vi "DisplayPanel.vi"() -> ()   [LabVIEW 2015]
uses:
  <vilib>/picture/picture.llb/imagedata.ctl
  MvLVLib/MvCameraControl.lvlib
panel:
  out "GenTLDevInfoArray":T1(array[cluster])
  out "GenTLIfInfoArray":T2(array[cluster])
  in  "Refresh Interaces":bool
  in  "Interface List":u16(ring) items=["[GenTL] GEVGenTL Interface Module"]
  in  "pConvertInfo In":T3
  out "PixelFormat":u32
  out "handle out":u64
  in  "handle":u64
  in  "Rectangle":T4
  in  "image data":T5 caption="图像数据"
  out "Picture":picture
  out "PayloadSize":u32
  out "pFrameInfoEx out":T6
  out "nHeight":u32
  out "nWidth":u32
  out "Acquisision Flag":bool
  in  "Trigger Mode":bool
  in  "Continuous":bool
  out "打开标志":bool
  in  "stop":bool
  in  "Trigger Once":bool
  in  "Stop":bool
  in  "Start":bool
  in  "Open Device":bool
  in  "Close Device":bool
  in  "error in (no error) 2":errorcluster caption="错误输入（无错误）"
  in  "Refresh Devices":bool
  in  "Device List":u16(ring) items=["[GenTL] DJFL MV-DB1608-05C-H-S(00202009042)", "[GenTL] SmartCamera_wmr MV-ID6089M-00C-NNG(00236610549)", "[GenTL] Don't Connect MV-CA013-20GM(00643989004)", "[GenTL] zyb MV-CA020-20GM(00683551272)", "[GenTL] 二维 MV-CA060-11GM(00815677386)", "[GenTL] ZLR MV-CE120-10GC(00C87836158)", "[GenTL] 132中文 MV-CA013-20GC(00C91585464)", "[GenTL] BionCamera1 MV-DB1308-05H(00D27684654)", "[GenTL] SZP 349Camera MV-ID6200M-00C-NNG(00D57564216)", "[GenTL] 8 MV-ID6200M-00C-NNG(00D75479067)", "[GenTL]  MV-DL2025-04H-H(00E35281809)", "[GenTL]  MV-DL2025-04H-H(00E47782357)", "[GenTL] smartcamera_ff MV-ID6200M-00C-NNG(00F36543614)", "[GenTL] left MV-ID6200M-00C-NNG(00F62465456)", "[GenTL]  EX-YTO-GM(00G02928059)", "[GenTL] BaseX86_1 MV-SI612-06GM(C12222347)", "[GenTL] CS060_csj MV-CS060-10GC-PRO(E55846631)", "[GenTL] zxc_SC_3016C MV-SC3016C-12M-WBN(G07812386)", "[GenTL] zxc_SC_2004EM MV-SC2004EM-06S-WBN(G32318424)"]
  # "Initialize"
  # "Acquisition"
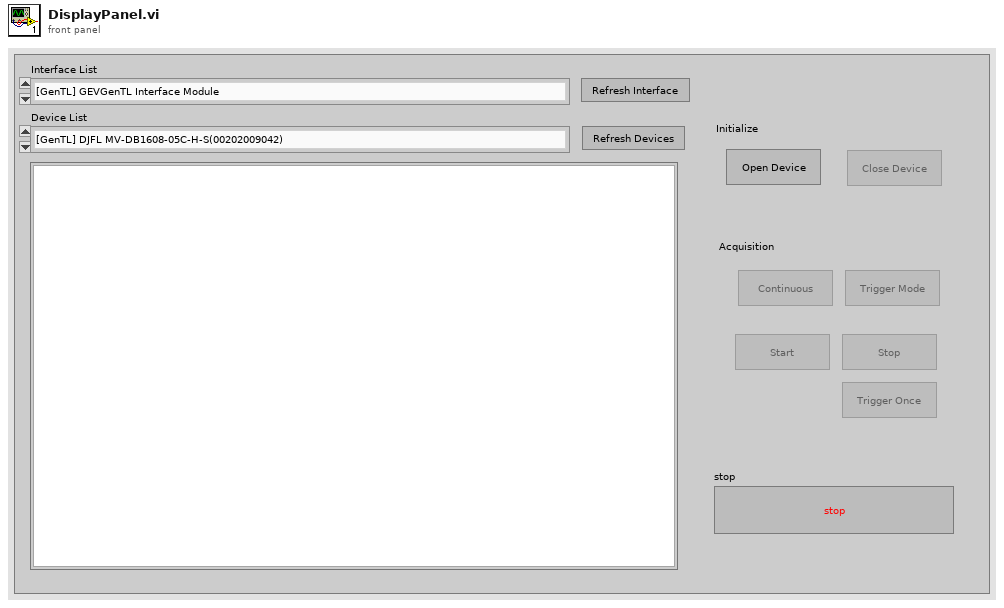
[diagram p1: front panel]
types:
  T1 = cluster{"chInterfaceID":string, "chDeviceID":string, "chVendorName":string, "chModelName":string, "chTLType":string, "chDisplayName":string, "chUserDefinedName":string, "chSerialNumber":string, "chDeviceVersion":string, "nCtiIndex":u32, "nReserved[0]":u32, "nReserved[1]":u32, "nReserved[2]":u32, "nReserved[3]":u32, "nReserved[4]":u32, "nReserved[5]":u32, "nReserved[6]":u32, "nReserved[7]":u32}[]
  T2 = cluster{"chInterfaceID":string, "chTLType":string, "chDisplayName":string, "nCtiIndex":u32, "nReserved[0]":u32, "nReserved[1]":u32, "nReserved[2]":u32, "nReserved[3]":u32, "nReserved[4]":u32, "nReserved[5]":u32, "nReserved[6]":u32, "nReserved[7]":u32}[]
  T3 = cluster{"nWidth":u16, "nHeight":u16, "enSrcPixelType":u32, "nSrcDataLen":u32, "enDstPixelType":u32, "nDstLen":u32, "nDstBufferSize":u32, "nRes0":u32, "nRes1":u32, "nRes2":u32, "nRes3":u32}
  T4 = cluster{"left":i16, "top":i16, "right":i16, "bottom":i16}
  T5 = typedef "imagedata.ctl" = cluster{"image type":i32, "image depth":i32, "image":u8[], "mask":u8[], "colors":u32[], "Rectangle":cluster{"left":i16, "top":i16, "right":i16, "bottom":i16}}
  T6 = cluster{"nWidth":u16, "nHeight":u16, "enPixelType":i32, "nFrameNum":u32, "nDevTimeStampHigh":u32, "nDevTimeStampLow":u32, "nReserved0":u32, "nHostTimeStamp":i64, "nFrameLen":u32, "nSecondCount]":u32, "nCycleCount":u32, "nCycleOffset":u32, "fGain":u32, "fExposureTime":u32, "nAverageBrightness":u32, "nRed":u32, "nGreen":u32, "nBlue":u32, "nFrameCounter":u32, "nTriggerIndex":u32, "nInput":u32, "nOutput":u32, "nOffsetX":u32, "nOffsetY":u32, "nReserved[0]":u32, "nReserved[1]":u32, "nReserved[2]":u32, "nReserved[3]":u32, "nReserved[4]":u32, "nReserved[5]":u32, "nReserved[6]":u32, "nReserved[7]":u32, "nReserved[8]":u32, "nReserved[9]":u32, "nReserved[10]":u32, "nReserved[11]":u32, "nReserved[12]":u32, "nReserved[13]":u32, "nReserved[14] 10":u32, "nReserved[15] 11":u32, "nReserved[16] 12":u32, "nReserved[17] 13":u32, "nReserved[18] 14":u32, "nReserved[19] 15":u32, "nReserved[20] 16":u32, "nReserved[21] 17":u32, "nReserved[22] 18":u32, "nReserved[23] 19":u32, "nReserved[24] 20":u32, "nReserved[25] 21":u32, "nReserved[26] 22":u32, "nReserved[27] 23":u32, "nReserved[28] 24":u32, "nReserved[29] 25":u32, "nReserved[30] 26":u32, "nReserved[31] 27":u32, "nReserved[32] 28":u32, "nReserved[33] 29":u32, "nReserved[34] 30":u32, "nReserved[35] 31":u32, "nReserved[36] 32":u32, "nReserved[37] 33":u32, "nReserved[38] 34":u32, "nReserved[39] 35":u32, "nReserved[40] 36":u32}
  T7 = enum8{"Enabled", "Disabled", "Disabled and Grayed Out"}
  T8 = cluster{"nCurValue":u32, "nMax":u32, "nMin":u32, "nInc":u32, "nReserved[0]":u32, "nReserved[1]":u32, "nReserved[2]":u32, "nReserved[3]":u32}
  T9 = cluster{"nCurValue":u32, "nSupportedNum":u32, "nSupportValue[0]":u32, "nSupportValue[1]":u32, "nSupportValue[2]":u32, "nSupportValue[3]":u32, "nSupportValue[4]":u32, "nSupportValue[5]":u32, "nSupportValue[6]":u32, "nSupportValue[7]":u32, "nSupportValue[8]":u32, "nSupportValue[9]":u32, "nSupportValue[10]":u32, "nSupportValue[11]":u32, "nSupportValue[12]":u32, "nSupportValue[13]":u32, "nSupportValue[14]":u32, "nSupportValue[15]":u32, "nSupportValue[16]":u32, "nSupportValue[17]":u32, "nSupportValue[18]":u32, "nSupportValue[19]":u32, "nSupportValue[20]":u32, "nSupportValue[21]":u32, "nSupportValue[22]":u32, "nSupportValue[23]":u32, "nSupportValue[24]":u32, "nSupportValue[25]":u32, "nSupportValue[26]":u32, "nSupportValue[27]":u32, "nSupportValue[28]":u32, "nSupportValue[29]":u32, "nSupportValue[30]":u32, "nSupportValue[31]":u32, "nSupportValue[32]":u32, "nSupportValue[33]":u32, "nSupportValue[34]":u32, "nSupportValue[35]":u32, "nSupportValue[36]":u32, "nSupportValue[37]":u32, "nSupportValue[38]":u32, "nSupportValue[39]":u32, "nSupportValue[40]":u32, "nSupportValue[41]":u32, "nSupportValue[42]":u32, "nSupportValue[43]":u32, "nSupportValue[44]":u32, "nSupportValue[45]":u32, "nSupportValue[46]":u32, "nSupportValue[47]":u32, "nSupportValue[48]":u32, "nSupportValue[49]":u32, "nSupportValue[50]":u32, "nSupportValue[51]":u32, "nSupportValue[52]":u32, "nSupportValue[53]":u32, "nSupportValue[54]":u32, "nSupportValue[55]":u32, "nSupportValue[56]":u32, "nSupportValue[57]":u32, "nSupportValue[58]":u32, "nSupportValue[59]":u32, "nSupportValue[60]":u32, "nSupportValue[61]":u32, "nSupportValue[62]":u32, "nSupportValue[63]":u32, "nReserved[0]":u32, "nReserved[1]":u32, "nReserved[2]":u32, "nReserved[3]":u32}
  T10 = cluster{"chInterfaceID":string, "chTLType":string, "chDisplayName":string, "nCtiIndex":u32, "nReserved[0]":u32, "nReserved[1]":u32, "nReserved[2]":u32, "nReserved[3]":u32, "nReserved[4]":u32, "nReserved[5]":u32, "nReserved[6]":u32, "nReserved[7]":u32}
  T11 = cluster{"chInterfaceID":string, "chDeviceID":string, "chVendorName":string, "chModelName":string, "chTLType":string, "chDisplayName":string, "chUserDefinedName":string, "chSerialNumber":string, "chDeviceVersion":string, "nCtiIndex":u32, "nReserved[0]":u32, "nReserved[1]":u32, "nReserved[2]":u32, "nReserved[3]":u32, "nReserved[4]":u32, "nReserved[5]":u32, "nReserved[6]":u32, "nReserved[7]":u32}
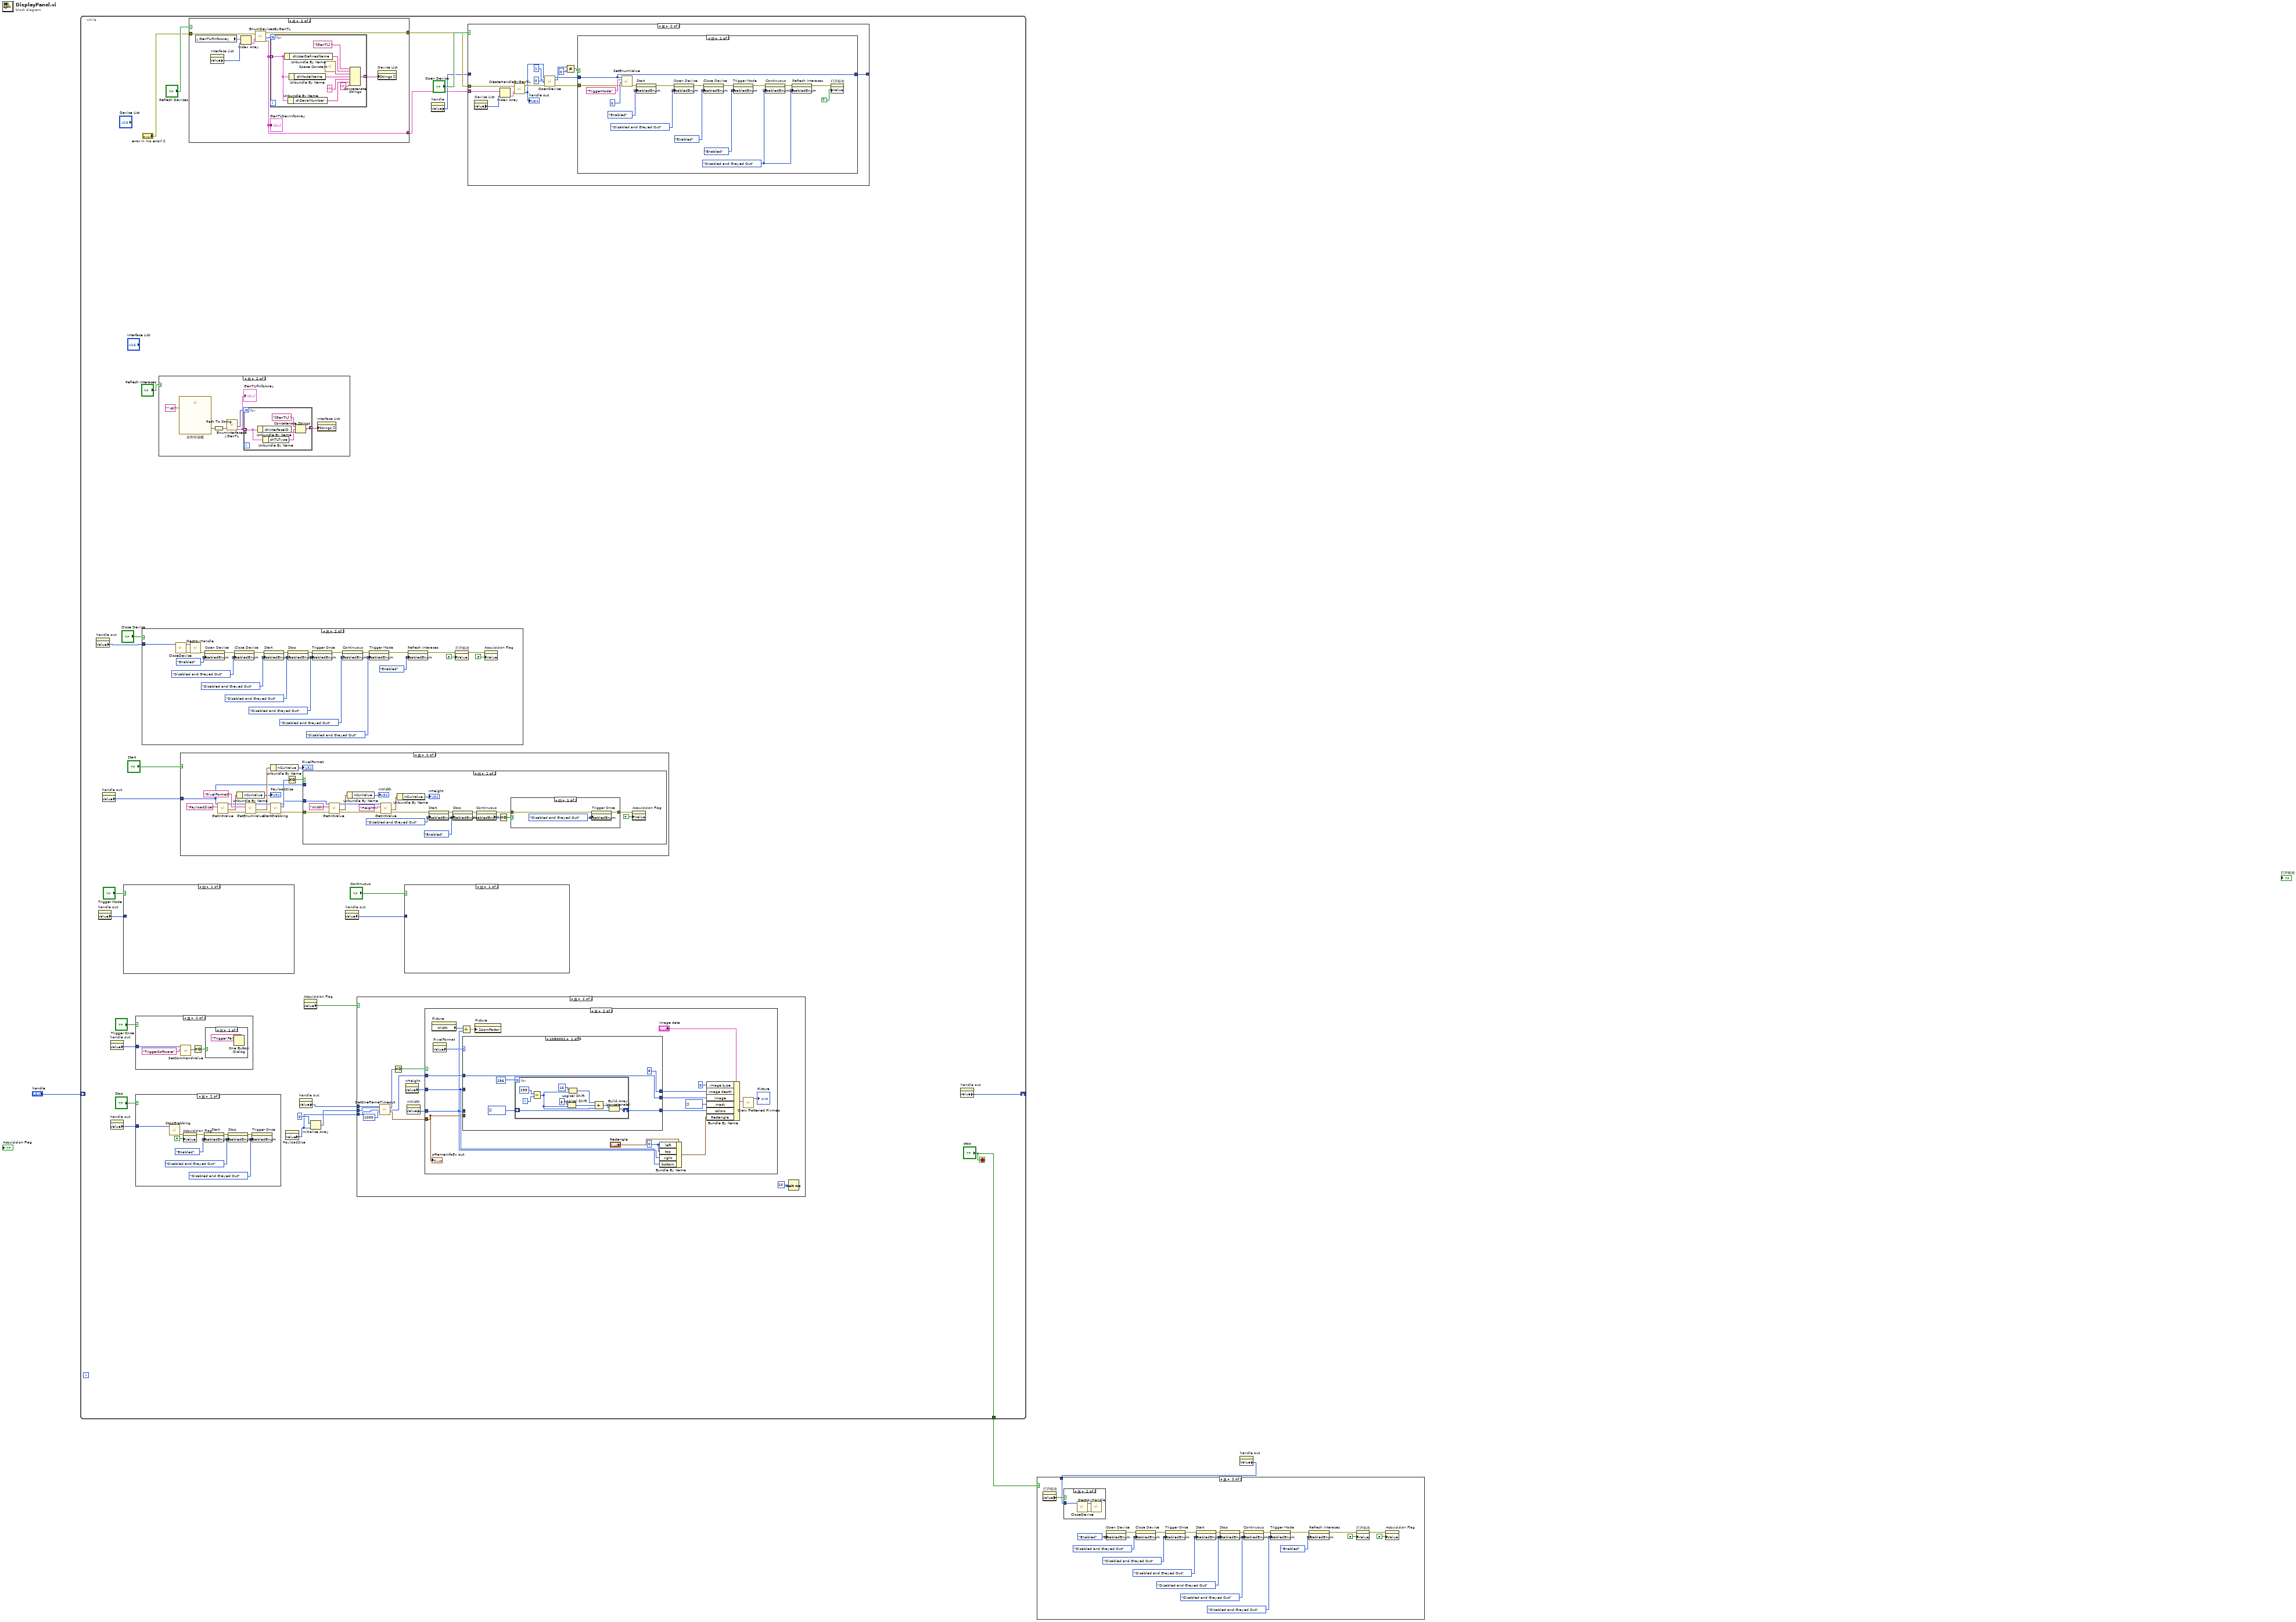
[diagram p0: block diagram]
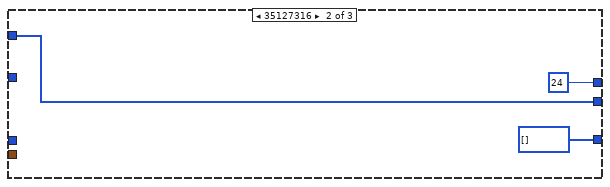
[diagram p7: hidden frame]
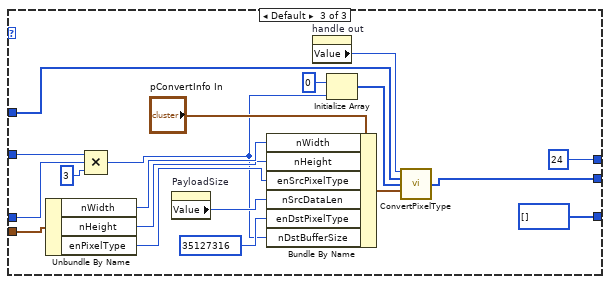
[diagram p8: hidden frame]
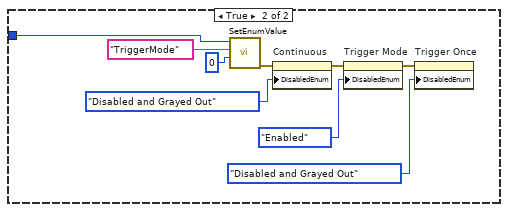
[diagram p10: hidden frame]
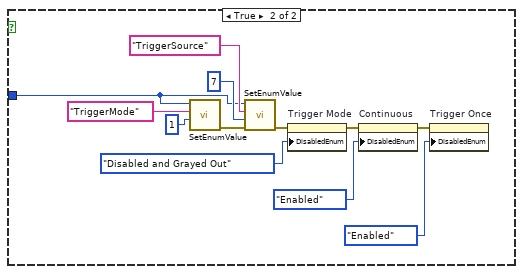
[diagram p11: hidden frame]
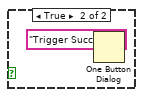
[diagram p13: hidden frame]
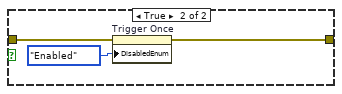
[diagram p15: hidden frame]
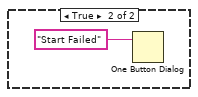
[diagram p16: hidden frame]
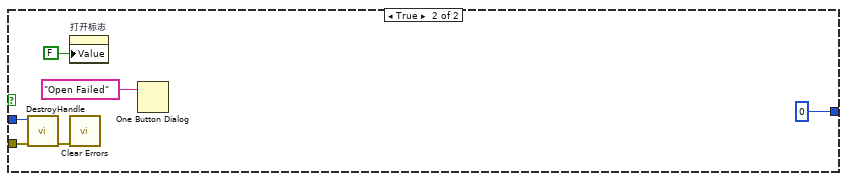
[diagram p19: hidden frame]
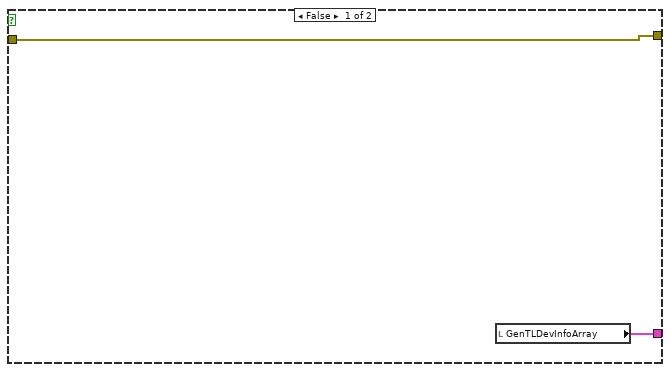
[diagram p20: hidden frame]
diagram:
  n1 = while {
    tunnel: ["stop"] -> w3
    shift-right: [w17] -> _
    shift-left: "handle" -> [_]
    stop <- "stop" stop-if-true
    n2 = property on="handle out" class="DigNum (严格)"() -> ("Value"=w15:u64)  [unwired: 2 in, 2 out]
    n3 = property on="handle out" class="DigNum (严格)"() -> ("Value"=w10:u64)  [unwired: 2 in, 2 out]
    n4 = property on="handle out" class="DigNum (严格)"() -> ("Value"=w11:u64)  [unwired: 2 in, 2 out]
    n5 = property on="handle out" class="DigNum (严格)"() -> ("Value"=w14:u64)  [unwired: 2 in, 2 out]
    n6 = property on="handle out" class="DigNum (严格)"() -> ("Value"=w13:u64)  [unwired: 2 in, 2 out]
    n7 = case shown="假" "Trigger Mode" {
      tunnel: w10 -> [_ w125]
      frame False {
      }
      frame True {
        n8 = call "SetEnumValue.vi"("nValue"=u32 1, "strKey"="TriggerMode", "handle"=w125) -> ("error out"=w131:errorcluster)  [unwired: 6 in, 2 out]
        n9 = call "SetEnumValue.vi"("error in (no error)"=w131, "nValue"=u32 7, "strKey"="TriggerSource", "handle"=w125) -> ("error out"=w130:errorcluster)  [unwired: 5 in, 2 out]
        n10 = property on="Trigger Mode" class="Bool"(error in=w130, "DisabledEnum"=T7."Disabled and Grayed Out" ("禁用")) -> (error out=w129:errorcluster)  [unwired: 1 in, 1 out]
        n11 = property on="Continuous" class="Bool"(error in=w129, "DisabledEnum"=T7."Enabled" ("禁用")) -> (error out=w127:errorcluster)  [unwired: 1 in, 1 out]
        n12 = property on="Trigger Once" class="Bool"(error in=w127, "DisabledEnum"=T7."Enabled" ("禁用")) -> ()  [unwired: 1 in, 2 out]
      }
    }
    n13 = case shown="真" "Trigger Once" {
      tunnel: w14 -> [_ w140]
      frame False {
      }
      frame True {
        n14 = call "SetCommandValue.vi"("strValue"="TriggerSoftware", "handle"=w140) -> ("function return"=w138:i32)  [unwired: 7 in, 2 out]
        n15 = Equal To 0?(x=w138) -> (x = 0?=w137:bool)
        n16 = case shown="假" w137 {
          frame False {
            n17 = One Button Dialog(message="Trigger Failed") -> ()  [unwired: 1 in, 1 out]
          }
          frame True {
            n18 = One Button Dialog(message="Trigger Success") -> ()  [unwired: 1 in, 1 out]
          }
        }
      }
    }
    n19 = case shown="真" "Stop" {
      tunnel: w13 -> [_ w115]
      frame False {
      }
      frame True {
        n20 = call "StopGrabbing.vi"("handle"=w115) -> ("error out"=w114:errorcluster)  [unwired: 8 in, 2 out]
        n21 = property on="Acquisision Flag" class="Bool (严格)"(error in=w114, "Value"=FALSE ("采集标志")) -> (error out=w109:errorcluster)  [unwired: 1 in, 1 out]
        n22 = property on="Start" class="Bool"(error in=w109, "DisabledEnum"=T7."Enabled" ("禁用")) -> (error out=w108:errorcluster)  [unwired: 1 in, 1 out]
        n23 = property on="Stop" class="Bool"(error in=w108, "DisabledEnum"=T7."Disabled and Grayed Out" ("禁用")) -> (error out=w107:errorcluster)  [unwired: 1 in, 1 out]
        n24 = property on="Trigger Once" class="Bool"(error in=w107, "DisabledEnum"=T7."Disabled and Grayed Out" ("禁用")) -> ()  [unwired: 1 in, 2 out]
      }
    }
    n25 = case shown="真" "Close Device" {
      tunnel: w15 -> [_ w190]
      frame False {
      }
      frame True {
        n26 = call "CloseDevice.vi"("handle"=w190) -> ("error out"=w192:errorcluster, "handle out"=w189:u64)  [unwired: 8 in, 1 out]
        n27 = call "DestroyHandle.vi"("error in (no error)"=w192, "handle"=w189) -> ("error out"=w191:errorcluster)  [unwired: 8 in, 1 out]
        n28 = property on="Open Device" class="Bool"(error in=w191, "DisabledEnum"=T7."Enabled" ("禁用")) -> (error out=w203:errorcluster)  [unwired: 1 in, 1 out]
        n29 = property on="Close Device" class="Bool"(error in=w203, "DisabledEnum"=T7."Disabled and Grayed Out" ("禁用")) -> (error out=w202:errorcluster)  [unwired: 1 in, 1 out]
        n30 = property on="Start" class="Bool"(error in=w202, "DisabledEnum"=T7."Disabled and Grayed Out" ("禁用")) -> (error out=w201:errorcluster)  [unwired: 1 in, 1 out]
        n31 = property on="Stop" class="Bool"(error in=w201, "DisabledEnum"=T7."Disabled and Grayed Out" ("禁用")) -> (error out=w200:errorcluster)  [unwired: 1 in, 1 out]
        n32 = property on="Trigger Once" class="Bool"(error in=w200, "DisabledEnum"=T7."Disabled and Grayed Out" ("禁用")) -> (error out=w197:errorcluster)  [unwired: 1 in, 1 out]
        n33 = property on="Continuous" class="Bool"(error in=w197, "DisabledEnum"=T7."Disabled and Grayed Out" ("禁用")) -> (error out=w196:errorcluster)  [unwired: 1 in, 1 out]
        n34 = property on="Trigger Mode" class="Bool"(error in=w196, "DisabledEnum"=T7."Disabled and Grayed Out" ("禁用")) -> (error out=w187:errorcluster)  [unwired: 1 in, 1 out]
        n35 = property on="Refresh Interaces" class="Bool"(error in=w187, "DisabledEnum"=T7."Enabled" ("禁用")) -> (error out=w186:errorcluster)  [unwired: 1 in, 1 out]
        n36 = property on="打开标志" class="Bool (严格)"(error in=w186, "Value"=FALSE ("打开标志")) -> (error out=w194:errorcluster)  [unwired: 1 in, 1 out]
        n37 = property on="Acquisision Flag" class="Bool (严格)"(error in=w194, "Value"=FALSE ("采集标志")) -> ()  [unwired: 1 in, 2 out]
      }
    }
    n38 = case shown="真" "Refresh Interaces" {
      frame False {
      }
      frame True {
        n39 = call "文件对话框"("pattern (all files)"="*.cti") -> ("selected path"=w34:path)  [unwired: 11 in, 3 out]
        n40 = Path To String(path=w34) -> (string=w33:string)
        n41 = call "EnumInterfacesByGenTL.vi"("strGenTLPath"=w33) -> ("nInterfaceNum"=w31:u32, "pGenTLIfInfoArray"=w32:T2)  [unwired: 1 in, 2 out]
        "GenTLIfInfoArray" <- w32
        n42 = for {
          N: w31 -> [_]
          tunnel: [w40] -> w30 mode=indexing
          tunnel: w32 -> [w37] mode=indexing
          n43 = Unbundle By Name(w37) -> ("chInterfaceID"=w38:string)
          n44 = Unbundle By Name(w37) -> ("chTLType"=w36:string)
          n45 = Concatenate Strings("[GenTL] " ("字符串"), w36, w38) -> (w40:string)
        }
        n46 = property on="Interface List" class="Ring (严格)"("Strings []"=w30) -> ()  [unwired: 2 in, 2 out]
      }
    }
    n47 = case shown="真" "Start" {
      tunnel: w11 -> [_ w147]
      frame False {
      }
      frame True {
        n48 = call "GetIntValue.vi"("strKey"="PayloadSize", "handle"=w147) -> ("error out"=w153:errorcluster, "pIntValue out"=w149:T8, "handle out"=w145:u64)  [unwired: 6 in, 1 out]
        n49 = Unbundle By Name(w149) -> ("nCurValue"=→"PayloadSize":u32)
        n50 = call "GetEnumValue.vi"("error in (no error)"=w153, "strKey"="PixelFormat", "handle"=w145) -> ("error out"=w152:errorcluster, "pEnumValue out"=w154:T9, "handle out"=w144:u64)  [unwired: 5 in, 1 out]
        n51 = Unbundle By Name(w154) -> ("nCurValue"=→"PixelFormat":u32)
        n52 = call "StartGrabbing.vi"("error in (no error)"=w152, "handle"=w144) -> ("error out"=w151:errorcluster, "function return"=w157:i32, "handle out"=w143:u64)  [unwired: 7 in]
        n53 = Not Equal To 0?(x=w157) -> (x != 0?=w156:bool)
        n54 = case shown="假" w156 {
          tunnel: w147 -> [_ _]
          tunnel: w151 -> [w160 _]
          tunnel: w143 -> [w159 _]
          frame False {
            n55 = call "GetIntValue.vi"("error in (no error)"=w160, "strKey"="Width", "handle"=w159) -> ("error out"=w167:errorcluster, "pIntValue out"=w161:T8, "handle out"=w158:u64)  [unwired: 5 in, 1 out]
            n56 = Unbundle By Name(w161) -> ("nCurValue"=→"nWidth":u32)
            n57 = call "GetIntValue.vi"("error in (no error)"=w167, "strKey"="Height", "handle"=w158) -> ("error out"=w166:errorcluster, "pIntValue out"=w164:T8)  [unwired: 5 in, 2 out]
            n58 = Unbundle By Name(w164) -> ("nCurValue"=→"nHeight":u32)
            n59 = property on="Start" class="Bool"(error in=w166, "DisabledEnum"=T7."Disabled and Grayed Out" ("禁用")) -> (error out=w176:errorcluster)  [unwired: 1 in, 1 out]
            n60 = property on="Stop" class="Bool"(error in=w176, "DisabledEnum"=T7."Enabled" ("禁用")) -> (error out=w162:errorcluster)  [unwired: 1 in, 1 out]
            n61 = property on="Continuous" class="Bool"(error in=w162) -> (error out=w172:errorcluster, "DisabledEnum"=w173:T7)  [unwired: 1 in, 1 out]
            n62 = Equal To 0?(x=w173) -> (x = 0?=w174:bool)
            n63 = case shown="假" w174 {
              tunnel: w172 -> [w179 w182]
              tunnel: [w178 w181] -> w171
              frame False {
                n64 = property on="Trigger Once" class="Bool"(error in=w179, "DisabledEnum"=T7."Disabled and Grayed Out" ("禁用")) -> (error out=w178:errorcluster)  [unwired: 1 in, 1 out]
              }
              frame True {
                n65 = property on="Trigger Once" class="Bool"(error in=w182, "DisabledEnum"=T7."Enabled" ("禁用")) -> (error out=w181:errorcluster)  [unwired: 1 in, 1 out]
              }
            }
            n66 = property on="Acquisision Flag" class="Bool (严格)"(error in=w171, "Value"=TRUE ("采集标志")) -> ()  [unwired: 1 in, 2 out]
          }
          frame True {
            n67 = One Button Dialog(message="Start Failed") -> ()  [unwired: 1 in, 1 out]
          }
        }
      }
    }
    n68 = case shown="真" "Refresh Devices" {
      tunnel: [w247 w250] -> w19
      tunnel: "error in (no error) 2" -> [w247 w251]
      tunnel: [w246 w248] -> w4
      frame False {
        n69 = local read "GenTLDevInfoArray"() -> (w246:T1)
      }
      frame True {
        n70 = local read "GenTLIfInfoArray"() -> (w253:T2)
        n71 = property on="Interface List" class="Ring (严格)"() -> ("Value"=w254:u16)  [unwired: 2 in, 2 out]
        n72 = Index Array(array=w253, index=w254) -> (element=w252:T10)
        n73 = call "EnumDevicesByGenTL.vi"("error in (no error)"=w251, "pIFInfo"=w252) -> ("error out"=w250:errorcluster, "nDeviceNum"=w249:u32, "pGenTLDevInfoArray"=w248:T1)  [unwired: 1 out]
        "GenTLDevInfoArray" <- w248
        n74 = for {
          N: w249 -> [_]
          tunnel: [w261] -> w255 mode=indexing
          tunnel: w248 -> [w259] mode=indexing
          n75 = Unbundle By Name(w259) -> ("chUserDefinedName"=w258:string)
          n76 = Unbundle By Name(w259) -> ("chSerialNumber"=w256:string)
          n77 = Unbundle By Name(w259) -> ("chModelName"=w257:string)
          n78 = call <vilib>:"Space Constant.vi"() -> ("String"=w264:string)
          n79 = Concatenate Strings("[GenTL] " ("字符串"), w258, w264, w257, "(" ("字符串"), w256, ")" ("字符串")) -> (w261:string)
        }
        n80 = property on="Device List" class="Ring (严格)"("Strings []"=w255) -> ()  [unwired: 2 in, 2 out]
      }
    }
    n81 = property on="PayloadSize" class="DigNum (严格)"() -> ("Value"=w6:u32)  [unwired: 2 in, 2 out]
    n82 = property on="handle out" class="DigNum (严格)"() -> ("Value"=w12:u64)  [unwired: 2 in, 2 out]
    n83 = property on="Acquisision Flag" class="Bool (严格)"() -> ("Value"=w21:bool)  [unwired: 2 in, 2 out]
    n84 = Initialize Array(u8 0 ("元素"), w6) -> (w7:u8[])
    n85 = property on="handle out" class="DigNum (严格)"() -> ("Value"=w9:u64)  [unwired: 2 in, 2 out]
    n86 = case shown="真" w21 {
      tunnel: w12 -> [_ w46]
      tunnel: w7 -> [_ w45]
      tunnel: w6 -> [_ w44]
      frame False {
      }
      frame True {
        n87 = call "GetOneFrameTimeout.vi"("handle"=w46, "pData"=w45, "nDataSize"=w44, "nMsec"=1000) -> ("function return"=w43:i32, "pData Out"=w42:u8[], "pFrameInfoEx out"=w41:T6)  [unwired: 7 in, 2 out]
        n88 = Equal To 0?(x=w43) -> (x = 0?=w50:bool)
        n89 = property on="nHeight" class="DigNum (严格)"() -> ("Value"=w48:u32)  [unwired: 2 in, 2 out]
        n90 = property on="nWidth" class="DigNum (严格)"() -> ("Value"=w49:u32)  [unwired: 2 in, 2 out]
        n91 = case shown="真" w50 {
          tunnel: w42 -> [_ w59]
          tunnel: w49 -> [_ w57]
          tunnel: w48 -> [_ w58]
          tunnel: w41 -> [_ w52]
          frame False {
          }
          frame True {
            w66 = i16 0 ("left")
            n92 = property on="Picture" class="Pict"() -> ("Width"=w61:u32)  [unwired: 2 in, 2 out]
            n93 = property on="PixelFormat" class="DigNum (严格)"() -> ("Value"=w53:u32)  [unwired: 2 in, 2 out]
            n94 = Divide(x=w61, y=w57) -> (x/y=w60:dbl)
            n95 = case shown="1080001" w53 {
              tunnel: w59 -> [w72 w87 w103]
              tunnel: w58 -> [_ _ w100]
              tunnel: w57 -> [_ _ w99]
              tunnel: [w72 w87 w88] -> w56
              tunnel: [8 24 24] -> w55
              tunnel: [w70 i32[] [] i32[] []] -> w54
              tunnel: w52 -> [_ _ w89]
              frame 17301505 {
                n96 = for {
                  N: 256 -> [_]
                  shift-right: [w79] -> w70
                  shift-left: i32[] [] ("数组") -> [w78]
                  i -> [w75]
                  n97 = Subtract(x=255, y=w75) -> (x-y=w76:i32)
                  n98 = Logical Shift(y=i16 8, x=w76) -> (x << y=w81:i32)
                  n99 = Logical Shift(y=16 ("x"), x=w76) -> (x << y=w82:i32)
                  n100 = Compound Arithmetic op=ADD(w82, w81, w76) -> (w80:i32)
                  n101 = Build Array (concatenate)(w80, w78) -> (w79:i32[])
                }
              }
              frame 35127316 {
              }
              frame Default {
                n102 = Unbundle By Name(w89) -> ("nWidth"=w98:u16, "nHeight"=w97:u16, "enPixelType"=w96:i32)
                n103 = Compound Arithmetic op=MULTIPLY(w100, w99, u32 3 ("值")) -> (w93:u32)
                n104 = property on="PayloadSize" class="DigNum (严格)"() -> ("Value"=w95:u32)  [unwired: 2 in, 2 out]
                n105 = Bundle By Name(cluster="pConvertInfo In", "nWidth"=w98, "nHeight"=w97, "enSrcPixelType"=w96, "nSrcDataLen"=w95, "enDstPixelType"=u32 35127316, "nDstBufferSize"=w93) -> (w92:T3)
                n106 = property on="handle out" class="DigNum (严格)"() -> ("Value"=w104:u64)  [unwired: 2 in, 2 out]
                n107 = Initialize Array(u8 0 ("元素"), w93) -> (w102:u8[])
                n108 = call "ConvertPixelType.vi"("handle"=w104, "pSrcData"=w103, "pDstBuf In"=w102, "pConvertInfo In"=w92) -> ("pDstBuf Out"=w88:u8[])  [unwired: 7 in, 4 out]
              }
            }
            n109 = property on="Picture" class="Pict"("ZoomFactor"=w60) -> ()  [unwired: 2 in, 2 out]
            n110 = Bundle By Name(cluster="Rectangle", "left"=w66, "top"=w66, "right"=w57, "bottom"=w58) -> (w63:T4)
            n111 = Bundle By Name(cluster="image data", "image type"=0, "image depth"=w55, "image"=w56, "mask"=u8[] [], "colors"=w54, "Rectangle"=w63) -> (w62:T5)
            n112 = call <vilib>:"Draw Flattened Pixmap.vi"("image data"=w62) -> ("new picture"=→"Picture":picture)  [unwired: 8 in]
            "pFrameInfoEx out" <- w52
          }
        }
        n113 = Wait (ms)(milliseconds to wait=u32 10 ("等待时间（毫秒）")) -> ()  [unwired: 1 out]
      }
    }
    n114 = case shown="假" "Continuous" {
      tunnel: w9 -> [_ w116]
      frame False {
      }
      frame True {
        n115 = call "SetEnumValue.vi"("nValue"=u32 0, "strKey"="TriggerMode", "handle"=w116) -> ("error out"=w117:errorcluster)  [unwired: 6 in, 2 out]
        n116 = property on="Continuous" class="Bool"(error in=w117, "DisabledEnum"=T7."Disabled and Grayed Out" ("禁用")) -> (error out=w121:errorcluster)  [unwired: 1 in, 1 out]
        n117 = property on="Trigger Mode" class="Bool"(error in=w121, "DisabledEnum"=T7."Enabled" ("禁用")) -> (error out=w119:errorcluster)  [unwired: 1 in, 1 out]
        n118 = property on="Trigger Once" class="Bool"(error in=w119, "DisabledEnum"=T7."Disabled and Grayed Out" ("禁用")) -> ()  [unwired: 1 in, 2 out]
      }
    }
    n119 = property on="handle" class="DigNum (严格)"() -> ("Value"=w16:u64)  [unwired: 2 in, 2 out]
    n120 = case shown="真" "Open Device" {
      tunnel: [w208 w217] -> _
      tunnel: w16 -> [w208 _]
      tunnel: w19 -> [_ w212]
      tunnel: w4 -> [_ w210]
      frame False {
      }
      frame True {
        n121 = property on="Device List" class="Ring (严格)"() -> ("Value"=w214:u16)  [unwired: 2 in, 2 out]
        n122 = Index Array(array=w210, index=w214) -> (element=w209:T11)
        n123 = call "CreateHandleByGenTL.vi"("error in (no error)"=w212, "pDevInfo"=w209) -> ("error out"=w213:errorcluster, "handle"=w211:u64)  [unwired: 1 out]
        "handle out" <- w211
        n124 = call "OpenDevice.vi"("error in (no error)"=w213, "nSwitchoverKey"=u16 0, "nAccessMode"=u32 1, "handle"=w211) -> ("error out"=w218:errorcluster, "return"=w216:i32, "handle out"=w215:u64)  [unwired: 5 in]
        n125 = Not Equal?(x=w216, y=0) -> (x != y?=w221:bool)
        n126 = case shown="假" w221 {
          tunnel: w215 -> [w226 w243]
          tunnel: w218 -> [w227 w240]
          tunnel: [w226 u64 0 ("handle")] -> w217
          frame False {
            w225 = T7."Disabled and Grayed Out" ("禁用")
            n127 = call "SetEnumValue.vi"("error in (no error)"=w227, "nValue"=u32 0, "strKey"="TriggerMode", "handle"=w226) -> ("error out"=w236:errorcluster)  [unwired: 5 in, 2 out]
            n128 = property on="Start" class="Bool"(error in=w236, "DisabledEnum"=T7."Enabled" ("禁用")) -> (error out=w234:errorcluster)  [unwired: 1 in, 1 out]
            n129 = property on="Open Device" class="Bool"(error in=w234, "DisabledEnum"=T7."Disabled and Grayed Out" ("禁用")) -> (error out=w233:errorcluster)  [unwired: 1 in, 1 out]
            n130 = property on="Close Device" class="Bool"(error in=w233, "DisabledEnum"=T7."Enabled" ("禁用")) -> (error out=w230:errorcluster)  [unwired: 1 in, 1 out]
            n131 = property on="Trigger Mode" class="Bool"(error in=w230, "DisabledEnum"=T7."Enabled" ("禁用")) -> (error out=w229:errorcluster)  [unwired: 1 in, 1 out]
            n132 = property on="Continuous" class="Bool"(error in=w229, "DisabledEnum"=w225) -> (error out=w224:errorcluster)  [unwired: 1 in, 1 out]
            n133 = property on="Refresh Interaces" class="Bool"(error in=w224, "DisabledEnum"=w225) -> (error out=w223:errorcluster)  [unwired: 1 in, 1 out]
            n134 = property on="打开标志" class="Bool (严格)"(error in=w223, "Value"=TRUE ("布尔")) -> ()  [unwired: 1 in, 2 out]
          }
          frame True {
            n135 = call "DestroyHandle.vi"("error in (no error)"=w240, "handle"=w243) -> ("error out"=w241:errorcluster)  [unwired: 8 in, 1 out]
            n136 = property on="打开标志" class="Bool (严格)"("Value"=FALSE) -> ()  [unwired: 2 in, 2 out]
            n137 = call <vilib>:"Clear Errors.vi"("error in (no error)"=w241) -> ()  [unwired: 5 in, 2 out]
            n138 = One Button Dialog(message="Open Failed") -> ()  [unwired: 1 in, 1 out]
          }
        }
      }
    }
    n139 = property on="handle out" class="DigNum (严格)"() -> ("Value"=w17:u64)  [unwired: 2 in, 2 out]
  }
  n140 = property on="handle out" class="DigNum (严格)"() -> ("Value"=w1:u64)  [unwired: 2 in, 2 out]
  n141 = case shown="真" w3 {
    tunnel: w1 -> [_ w280]
    frame False {
    }
    frame True {
      n142 = property on="打开标志" class="Bool (严格)"() -> ("Value"=w271:bool)  [unwired: 2 in, 2 out]
      n143 = case shown="真" w271 {
        tunnel: w280 -> [_ w287]
        frame False {
        }
        frame True {
          n144 = call "CloseDevice.vi"("handle"=w287) -> ("error out"=w288:errorcluster, "handle out"=w286:u64)  [unwired: 8 in, 1 out]
          n145 = call "DestroyHandle.vi"("error in (no error)"=w288, "handle"=w286) -> ()  [unwired: 8 in, 2 out]
        }
      }
      n146 = property on="Open Device" class="Bool"("DisabledEnum"=T7."Enabled" ("禁用")) -> (error out=w279:errorcluster)  [unwired: 2 in, 1 out]
      n147 = property on="Close Device" class="Bool"(error in=w279, "DisabledEnum"=T7."Disabled and Grayed Out" ("禁用")) -> (error out=w278:errorcluster)  [unwired: 1 in, 1 out]
      n148 = property on="Trigger Once" class="Bool"(error in=w278, "DisabledEnum"=T7."Disabled and Grayed Out" ("禁用")) -> (error out=w277:errorcluster)  [unwired: 1 in, 1 out]
      n149 = property on="Start" class="Bool"(error in=w277, "DisabledEnum"=T7."Disabled and Grayed Out" ("禁用")) -> (error out=w276:errorcluster)  [unwired: 1 in, 1 out]
      n150 = property on="Stop" class="Bool"(error in=w276, "DisabledEnum"=T7."Disabled and Grayed Out" ("禁用")) -> (error out=w275:errorcluster)  [unwired: 1 in, 1 out]
      n151 = property on="Continuous" class="Bool"(error in=w275, "DisabledEnum"=T7."Disabled and Grayed Out" ("禁用")) -> (error out=w273:errorcluster)  [unwired: 1 in, 1 out]
      n152 = property on="Trigger Mode" class="Bool"(error in=w273, "DisabledEnum"=T7."Disabled and Grayed Out" ("禁用")) -> (error out=w266:errorcluster)  [unwired: 1 in, 1 out]
      n153 = property on="Refresh Interaces" class="Bool"(error in=w266, "DisabledEnum"=T7."Enabled" ("禁用")) -> (error out=w265:errorcluster)  [unwired: 1 in, 1 out]
      n154 = property on="打开标志" class="Bool (严格)"(error in=w265, "Value"=FALSE ("打开标志")) -> (error out=w268:errorcluster)  [unwired: 1 in, 1 out]
      n155 = property on="Acquisision Flag" class="Bool (严格)"(error in=w268, "Value"=FALSE ("采集标志")) -> ()  [unwired: 1 in, 2 out]
    }
  }
